vi "MGI Default ini Path.vi"(8 "File Extension (.ini)":string=".ini", 9 "All Users? (True)":bool=TRUE, 10 "File Name (Caller's Prefix)":string, 11 "Folder Name (Caller's Prefix)":string) -> (3 "Path":path)   [LabVIEW 2016]
doc: "This VI constructs a standardized configuration file path in either MyDocuments or All Users\\Documents depending on \"All Users?\". \n\n\n\nAuthored by Robert C. Mortensen\nsupport@mooregoodideas.com\nwww.mooregoodideas.com\n\nCopyright (c) 2010, Moore Good Ideas, Inc.\n\nAll rights reserved.\n\nRedistribution and use in source and binary forms, with or without modification, are permitted provided that the following conditions are met:\n\n * Redistributions of source code must retain the above copyright notice, this list of conditions and the following disclaimer.\n * Redistributions in binary form must reproduce the above copyright notice, this list of conditions and the following disclaimer in the documentation and/or other materials provided with the distribution.\n * Neither the name of Moore Good Ideas, Inc. nor the names of its contributors may be used to endorse or promote products derived from this software without specific prior written permission.\n\nTHIS SOFTWARE IS PROVIDED BY THE COPYRIGHT HOLDERS AND CONTRIBUTORS \"AS IS\" AND ANY EXPRESS OR IMPLIED WARRANTIES, INCLUDING, BUT NOT LIMITED TO, THE IMPLIED WARRANTIES OF MERCHANTABILITY AND FITNESS FOR A PARTICULAR PURPOSE ARE DISCLAIMED. IN NO EVENT SHALL THE COPYRIGHT OWNER OR CONTRIBUTORS BE LIABLE FOR ANY DIRECT, INDIRECT, INCIDENTAL, SPECIAL, EXEMPLARY, OR CONSEQUENTIAL DAMAGES (INCLUDING, BUT NOT LIMITED TO, PROCUREMENT OF SUBSTITUTE GOODS OR SERVICES; LOSS OF USE, DATA, OR PROFITS; OR BUSINESS INTERRUPTION) HOWEVER CAUSED AND ON ANY THEORY OF LIABILITY, WHETHER IN CONTRACT, STRICT LIABILITY, OR TORT (INCLUDING NEGLIGENCE OR OTHERWISE) ARISING IN ANY WAY OUT OF THE USE OF THIS SOFTWARE, EVEN IF ADVISED OF THE POSSIBILITY OF SUCH DAMAGE."
uses:
  <userlib>/_MGI/File/MGI Create Directory Chain Behavior Enum.ctl
  <userlib>/_MGI/File/MGI Windows Folder Enum.ctl
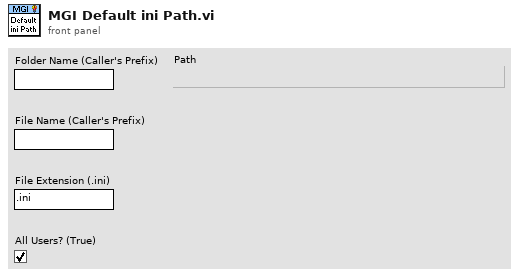
[diagram p1: front panel]
types:
  T1 = typedef "MGI Create Directory Chain Behavior Enum.ctl" = enum16{"Auto Detect", "Path Contains a File", "Path Does Not Contain a File"}
  T2 = typedef "MGI Windows Folder Enum.ctl" = enum32{"Desktop", "Err<Internet>", "Programs", "Err<Controls>", "Err<Printers>", "Personal (MyDocuments)", "Favorites", "Startup", "Recent", "SendTo", "Err<RecycleBin>", "StartMenu", "Err<MyDocuments>", "MyMusic", "MyVideo", "Err<0x000F>", "DesktopDirectory", "Err<Drives>", "Err<Network>", "NetHood", "Fonts", "Templates", "CommonStartMenu", "CommonPrograms", "CommonStartup", "CommonDesktopDirectory", "AppData", "PrintHood", "LocalAppData", "Err<AltStartup>", "Err<CommonAltStartup>", "CommonFavorites", "InternetCache", "Cookies", "History", "CommonAppData", "Windows", "System", "ProgramFiles", "MyPictures", "Profile", "System32", "Err<0x002A>", "ProgramFilesCommon", "Err<0x002C>", "CommonTemplates", "CommonDocuments", "CommonAdminTools", "AdminTools"}
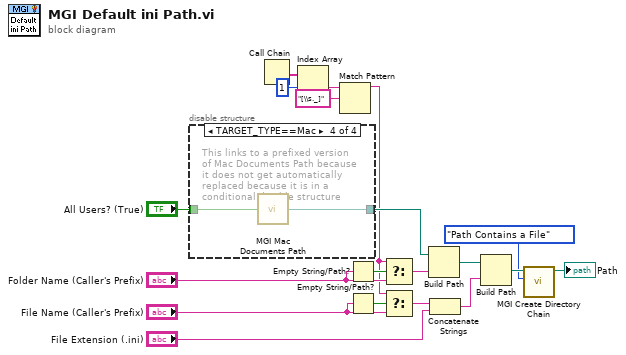
[diagram p0: block diagram]
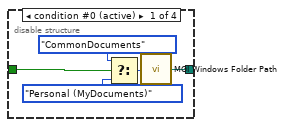
[diagram p2: hidden frame]
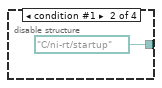
[diagram p3: hidden frame]
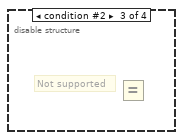
[diagram p4: hidden frame]
diagram:
  n1 = disable-structure shown="TARGET_TYPE==Mac" {
    disable-tunnel: [w24 path "C:/ni-rt/startup" ("Path") _ w26] -> w17
    disable-tunnel: "All Users? (True)" -> [w20 _ _ w27]
    frame condition #0 (active) {
      n2 = Select(t=MGI_Windows_Folder_Enum."CommonDocuments" ("Special Folder"), s=w20, f=MGI_Windows_Folder_Enum."Personal (MyDocuments)" ("Special Folder")) -> (s? t:f=w21:T2)
      n3 = call <userlib>:"MGI Windows Folder Path.vi"("Windows Folder"=w21) -> ("Path"=w24:path)
    }
    frame condition #1 {
    }
    frame condition #2 {
      # "Not supported"
      n4 = Equal?() -> ()  [unwired: 2 in, 1 out]
    }
    frame condition #3 {
      # "This links to a prefixed version of Mac Documents Path because it does not get automatically replaced because it is in a conditional disable structure"
      n5 = call <userlib>:"MGI Mac Documents Path.vi"("User Documents? (F: Shared Documents)"=w27) -> ("Path"=w26:path)
    }
  }
  n6 = Call Chain() -> (call chain=w9:string[])
  n7 = Index Array(array=w9, index=1) -> (element=w10:string)
  n8 = Match Pattern(string=w10, regular expression="[\\s._]") -> (before substring=w4:string)  [unwired: 1 in, 3 out]
  n9 = Empty String/Path?(string/path="Folder Name (Caller's Prefix)") -> (empty?=w8:bool)
  n10 = Empty String/Path?(string/path="File Name (Caller's Prefix)") -> (empty?=w5:bool)
  n11 = Select(t=w4, s=w8, f="Folder Name (Caller's Prefix)") -> (s? t:f=w6:string)
  n12 = Select(t=w4, s=w5, f="File Name (Caller's Prefix)") -> (s? t:f=w2:string)
  n13 = Build Path(base path=w17, name or relative path=w6) -> (appended path=w16:path)
  n14 = Concatenate Strings(w2, "File Extension (.ini)") -> (w19:string)
  n15 = Build Path(base path=w16, name or relative path=w19) -> (appended path=w14:path)
  n16 = call <userlib>:"MGI Create Directory Chain.vi"("File Presence (Auto Detect)"=MGI_Create_Directory_Chain_Behavior_Enum."Path Contains a File", "Path"=w14) -> ("Duplicate Path"=→"Path":path)  [unwired: 8 in, 1 out]
